vi "Read_Timestamp_from_Text.vi"(8 "error in (no error)":errorcluster, 11 "Txt File path":path) -> (0 "error out":errorcluster, 2 "Number of timestamps":i32, 3 "relative timestamp (ns)":u64[](array[numeric]))   [LabVIEW 2020]
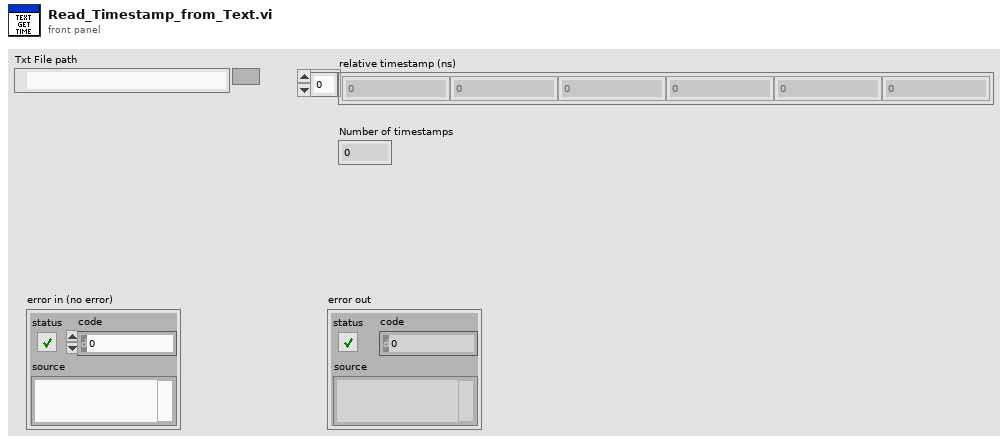
[diagram p1: front panel]
types:
  T1 = enum16{"open", "replace", "create", "open or create", "replace or create", "replace or create with confirmation"}
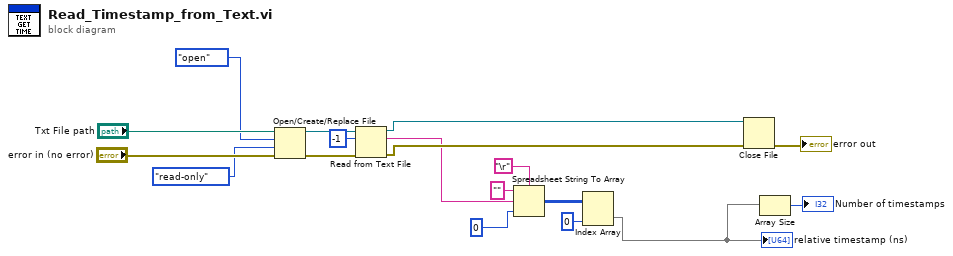
[diagram p0: block diagram]
diagram:
  n1 = Open/Create/Replace File(file path (use dialog)="Txt File path", error in="error in (no error)", operation (0:open)=T1."open", access (0:read/write)=enum16{"read/write", "read-only", "write-only"}."read-only") -> (refnum out=w12:refnum<file>, error out=w13:errorcluster)  [unwired: 2 in, 1 out]
  n2 = Read from Text File(file (use dialog)=w12, count=-1, error in=w13) -> (refnum out=w10:refnum<file>, text=w7:string, error out=w9:errorcluster)  [unwired: 1 in, 1 out]
  n3 = Spreadsheet String To Array(delimiter (Tab)="\r", format string="", spreadsheet string=w7, array type (2D Dbl)=u64 0) -> (array=w3:u64[][])
  n4 = Index Array(array=w3, index (col)=0 ("disabled index (col)")) -> (element=w2:u64[])  [unwired: 1 in]
  "relative timestamp (ns)" <- w2
  n5 = Close File(refnum=w10, error in=w9) -> (error out=→"error out":errorcluster)  [unwired: 1 out]
  n6 = Array Size(array=w2) -> (size(s)=→"Number of timestamps":i32)
